vi "LIDAR Global.vi"() -> ()   [LabVIEW 2014]
panel:
  out "I2C LIDAR":bool
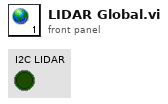
[diagram p1: front panel]
diagram:
